vi "Get Values.vi"(8 "error in (no error)":errorcluster, 11 "Object Entry in":refnum<class "Section.lvclass">) -> (0 "error out":errorcluster, 2 "Values":string[](array[string]), 3 "Object Entry out":refnum<class "Section.lvclass">)   [LabVIEW 2024, in "EDS.lvlib" / "Section.lvclass"]
uses:
  Section.lvclass
  Section.lvclass/Section.ctl
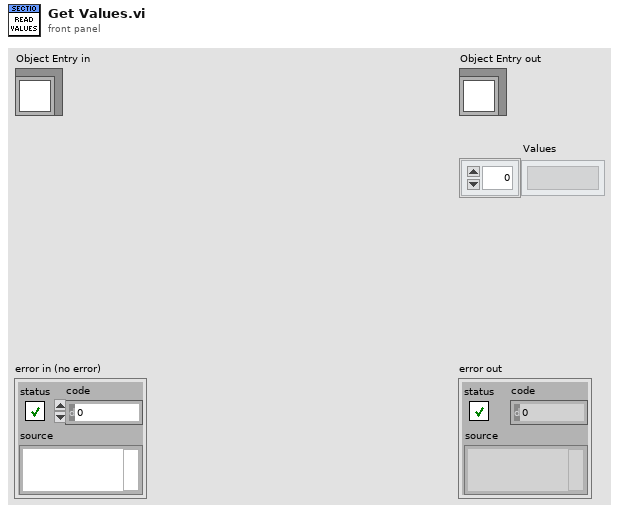
[diagram p1: front panel]
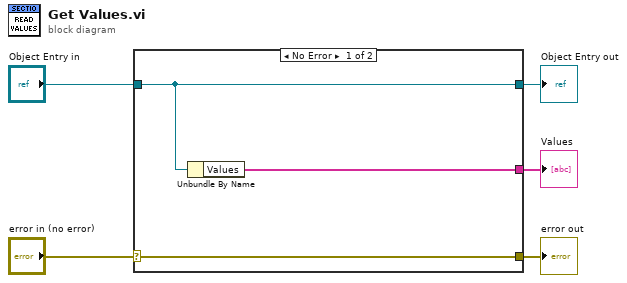
[diagram p0: block diagram]
diagram:
  n1 = case shown="No Error" "error in (no error)" {
    selector: "error in (no error)" -> [w8 w9]
    tunnel: [w8 w9] -> w4
    tunnel: [w7 w10] -> w2
    tunnel: "Object Entry in" -> [w7 w10]
    tunnel: [w6 _] -> w1
    frame No Error {
      n2 = Unbundle By Name(w7) -> ("Values"=w6:string[])
    }
    frame Error {
    }
  }
  "error out" <- w4
  "Object Entry out" <- w2
  "Values" <- w1
